vi "Signal FPGA to start acquisition.vi"(8 "error in (no error)":errorcluster, 10 "Logging queue element":T2={"Imaging Protocol"=enum."Live Imaging", "Number of Trials"=0, "Frame Size"=512, "# Averaged frames"=0, "Dwell time (us)"=0.0, "Index of Z-plane"=0, "Timelapse?"=FALSE, "Logging process is active"=FALSE, "Speed logging enabled"=FALSE, "tdms file ref"=refnum, "path"=path "", "Trial Number"=0, "Expected # points acquired"=FALSE, "Manually stopped"=FALSE, "Last trial"=FALSE, "Ch0 data"=[], "Ch1 data"=[], "Ref Data"=[], "Ref Frame Time"=[], "Image Time"=[], "Continuous Time"=[], "Ref X Length"=0, "Ref Y Length"=0, "# Ref Averaged frames"=0, "Ref Dwell time (us)"=0.0, "Points acquired"={"Ch0 last trial"=0, "Ch1 last trial"=0, "All trials"=0}, "HW Timings File"=refnum} {"Ref Dwell time (us)" format="%#.6g"; "Frame Size" items=["100X100"=100, "128X128"=128, "200X200"=200, "256X256"=256, "512X512"=512, "1024x1024"=1024, "2048x2048"=2048]; "Dwell time (us)" format="%#.6g"}, 11 "FPGA VI Ref":T1) -> (0 "error out":errorcluster, 3 "FPGA VI Reference Out":T1)   [LabVIEW 2017]
uses:
  RIG-SPECIFIC FILES/FPGA Refs/FPGA Ref.ctl
  Typedefs/Logging queue element.ctl
  Typedefs/Imaging Protocols enum.ctl
  Typedefs/Frame Size.ctl
  Typedefs/Acquired points count.ctl
  <vilib>/Utility/error.llb/Error Cluster From Error Code.vi
  <vilib>/rvi/errors/niLvFpgaAdjustHostInterfaceError.vi
  Global Variables/General Globals.vi
  <vilib>/rvi/interface/nirviReadWriteControl/nirviReadWriteControl.xnode
  NiFpgaLv.dll
  <vilib>/rvi/interface/Simulation/niFpgaSimulationCallBeginRW.vi
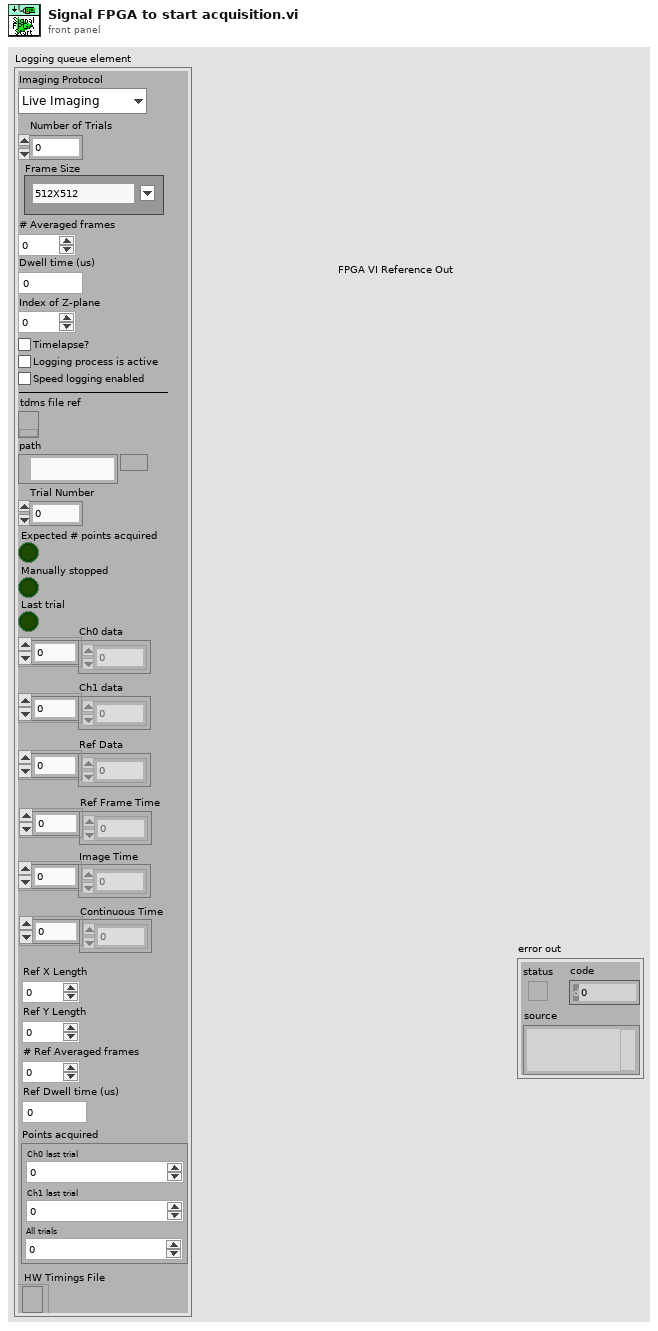
[diagram p1: front panel]
types:
  T1 = typedef "FPGA Ref.ctl" = refnum<k20>
  T2 = typedef "Logging queue element.ctl" = cluster{"Imaging Protocol":T3, "Number of Trials":u16, "Frame Size":T4, "# Averaged frames":u16, "Dwell time (us)":dbl, "Index of Z-plane":i32, "Timelapse?":bool, "Logging process is active":bool, "Speed logging enabled":bool, "tdms file ref":refnum<k34>, "path":path, "Trial Number":i32, "Expected # points acquired":bool, "Manually stopped":bool, "Last trial":bool, "Ch0 data":u32[], "Ch1 data":u32[], "Ref Data":u32[], "Ref Frame Time":u64[], "Image Time":u64[], "Continuous Time":u64[], "Ref X Length":u16, "Ref Y Length":u16, "# Ref Averaged frames":u16, "Ref Dwell time (us)":dbl, "Points acquired":T5, "HW Timings File":refnum<file>}
  T3 = typedef "Imaging Protocols enum.ctl" = enum16{"AOL Z-Stack", "Motor Z Stack", "Functional Acquisition", "Single Plane Acquisition", "Volume Acquisition", "Live Imaging", "Live Plane Imaging", "Live Volume Imaging"}
  T4 = typedef "Frame Size.ctl" = u16
  T5 = typedef "Acquired points count.ctl" = cluster{"Ch0 last trial":u64, "Ch1 last trial":u64, "All trials":u64}
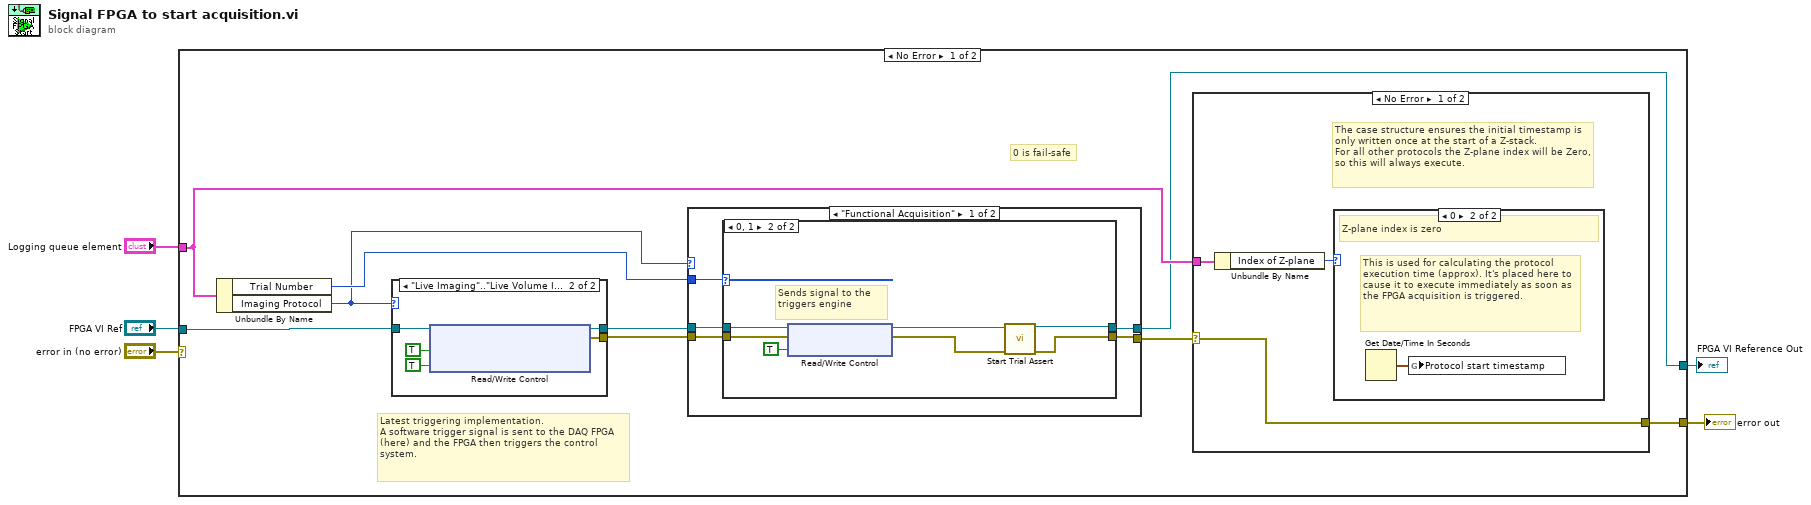
[diagram p0: block diagram]
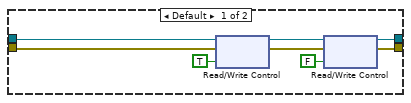
[diagram p2: hidden frame]
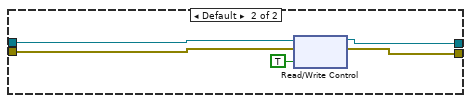
[diagram p3: hidden frame]
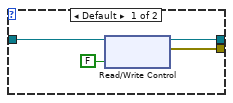
[diagram p6: hidden frame]
diagram:
  n1 = case shown="No Error" "error in (no error)" {
    selector: "error in (no error)" -> [_ w55]
    tunnel: [w13 w55] -> w5
    tunnel: "FPGA VI Ref" -> [w14 w54]
    tunnel: "Logging queue element" -> [w12 _]
    tunnel: [w8 w54] -> w1
    frame No Error {
      # "0 is fail-safe"
      # "Latest triggering implementation.\nA software trigger signal is sent to the DAQ FPGA (here) and the FPGA then triggers the control system."
      n2 = Unbundle By Name(w12) -> ("Trial Number"=w11:i32, "Imaging Protocol"=w10:T3)
      n3 = case shown="\"Live Imaging\"..\"Live Volume Imaging\"" w10 {
        tunnel: w14 -> [w47 w53]
        tunnel: [w46 w52] -> w7
        tunnel: [w45 w50] -> w6
        frame Default {
          n4 = xnode "Read/Write Control"("FPGA VI Reference In"=w47, "live_scan"=FALSE) -> ("FPGA VI Reference Out"=w46:T1, "error out"=w45:errorcluster)  [unwired: 1 in]
        }
        frame "Live Imaging".."Live Volume Imaging" {
          n5 = xnode "Read/Write Control"("FPGA VI Reference In"=w53, "live_scan"=TRUE, "live_scan (triggers module)"=TRUE) -> ("FPGA VI Reference Out"=w52:T1, "error out"=w50:errorcluster)  [unwired: 1 in]
        }
      }
      n6 = case shown="\"Functional Acquisition\"" w10 {
        tunnel: w7 -> [w15 w38]
        tunnel: w6 -> [w16 w37]
        tunnel: [w18 w36] -> w8
        tunnel: [w17 w35] -> w9
        tunnel: w11 -> [w19 _]
        frame "Functional Acquisition" {
          n7 = case shown="0, 1" w19 {
            tunnel: w15 -> [w26 w32]
            tunnel: [w23 w34] -> w18
            tunnel: w16 -> [w25 w31]
            tunnel: [w20 w33] -> w17
            frame Default {
              n8 = xnode "Read/Write Control"("FPGA VI Reference In"=w26, "error in"=w25, "start"=TRUE) -> ("FPGA VI Reference Out"=w22:T1, "error out"=w21:errorcluster)
              n9 = xnode "Read/Write Control"("FPGA VI Reference In"=w22, "error in"=w21, "start"=FALSE) -> ("FPGA VI Reference Out"=w23:T1, "error out"=w20:errorcluster)
            }
            frame 0, 1 {
              # "Sends signal to the triggers engine"
              n10 = xnode "Read/Write Control"("FPGA VI Reference In"=w32, "error in"=w31, "Experiment start"=TRUE ("start")) -> ("FPGA VI Reference Out"=w30:T1, "error out"=w29:errorcluster)
              n11 = call "Start Trial Assert.vi"("error in"=w29, "FPGA VI Ref"=w30) -> ("error out"=w33:errorcluster, "FPGA VI Reference Out"=w34:T1)  [unwired: 8 in]
            }
          }
        }
        frame Default {
          n12 = xnode "Read/Write Control"("FPGA VI Reference In"=w38, "error in"=w37, "start"=TRUE) -> ("FPGA VI Reference Out"=w36:T1, "error out"=w35:errorcluster)
        }
      }
      n13 = case shown="No Error" w9 {
        selector: w9 -> [w42 w44]
        tunnel: [w42 w44] -> w13
        tunnel: w12 -> [w41 _]
        frame No Error {
          # "The case structure ensures the initial timestamp is only written once at the start of a Z-stack.\nFor all other protocols the Z-plane index will be Zero, so this will always execute."
          n14 = Unbundle By Name(w41) -> ("Index of Z-plane"=w40:i32)
          n15 = case shown="0" w40 {
            frame Default {
              # "Z-plane index is other than zero"
            }
            frame 0 {
              # "This is used for calculating the protocol execution time (approx). It's placed here to cause it to execute immediately as soon as the FPGA acquisition is triggered."
              # "Z-plane index is zero"
              n16 = Get Date/Time In Seconds() -> (seconds since 1Jan1904=w43:timestamp)
              n17 = global write "General Globals.vi" "Protocol start timestamp"(w43) -> ()
            }
          }
        }
        frame Error {
        }
      }
    }
    frame Error {
    }
  }
  "error out" <- w5
  "FPGA VI Reference Out" <- w1
